vi "Circle dia adjust.vi"(8 "error in (no error)":errorcluster, 9 "Inspection \nmode?":bool, 10 "Cluster in":T1, 11 "Image in":T2) -> (0 "error out":errorcluster, 1 "Overlay Coordinates":cluster{"X":sgl, "Y":sgl}[](array[cluster]), 2 "Text origin":cluster{"X":sgl, "Y":sgl}, 3 "Image out":T2)   [LabVIEW 2019]
uses:
  <vilib>/vision/Image Controls.llb/IMAQ Image.ctl
  Controls/Circle dia data.ctl
  <vilib>/vision/NI_Vision_Development_Module.lvlib
panel:
  out "Angle":sgl
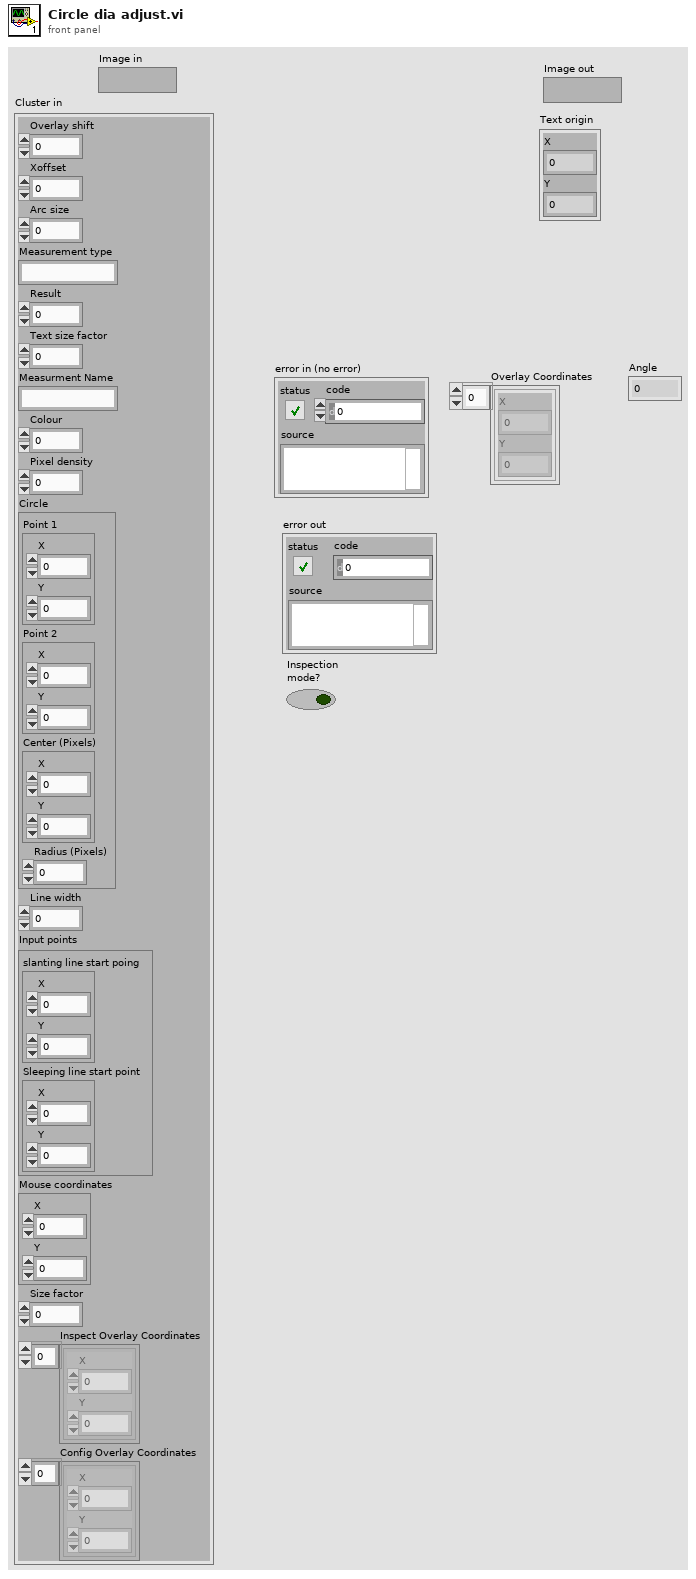
[diagram p1: front panel]
types:
  T1 = typedef "Circle dia data.ctl" = cluster{"Overlay shift":dbl, "Xoffset":i32, "Arc size":dbl, "Measurement type":string, "Result":sgl, "Text size factor":u32, "Measurment Name":string, "Colour":u32, "Pixel density":dbl, "Circle":cluster{"Point 1":cluster{"X":sgl, "Y":sgl}, "Point 2":cluster{"X":sgl, "Y":sgl}, "Center (Pixels)":cluster{"X":sgl, "Y":sgl}, "Radius (Pixels)":dbl}, "Line width":i32, "Input points":cluster{"slanting line start poing":cluster{"X":sgl, "Y":sgl}, "Sleeping line start point":cluster{"X":sgl, "Y":sgl}}, "Mouse coordinates":cluster{"X":sgl, "Y":sgl}, "Size factor":sgl, "Inspect Overlay Coordinates":cluster{"X":sgl, "Y":sgl}[], "Config Overlay Coordinates":cluster{"X":sgl, "Y":sgl}[]}
  T2 = typedef "IMAQ Image.ctl" = refnum<image>
  T3 = cluster{"Desired Font (Application)":enum16{"User-specified Font", "Application Font", "System Font", "Dialog Font"}, "[User-specified Font]":cluster{"Font Name":string, "Size":i16, "Strikeout?":bool, "Italic?":bool, "Underline?":bool, "Outline?":bool, "Shadow?":bool, "Bold?":bool, "Rotation Angle":dbl}, "Horizontal Alignment":i16, "Vertical Alignment":i16}
  T4 = cluster{"Left":i32, "Top":i32, "Right":i32, "Bottom":i32}
  T5 = cluster{"Point 1":cluster{"X":sgl, "Y":sgl}, "Point 2":cluster{"X":sgl, "Y":sgl}, "Center (Pixels)":cluster{"X":sgl, "Y":sgl}, "Radius (Pixels)":dbl}
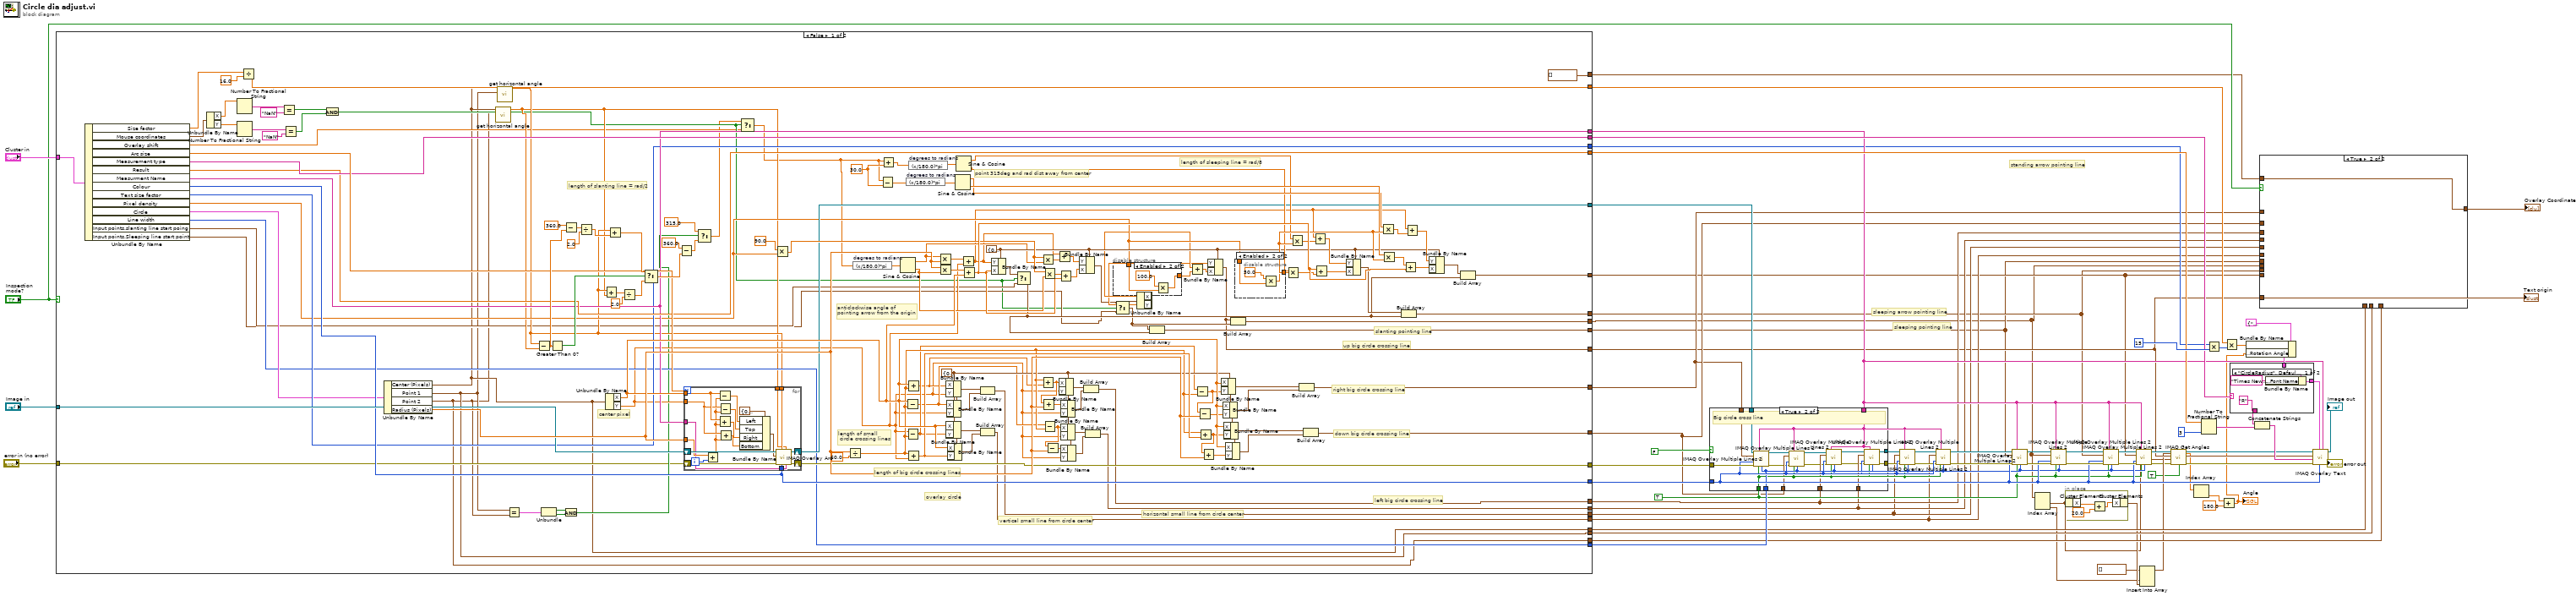
[diagram p0: block diagram]
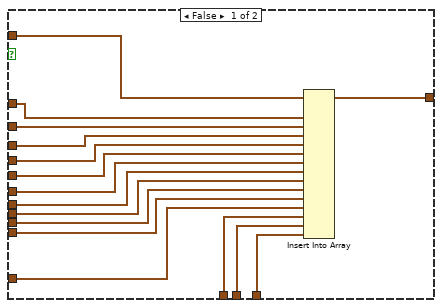
[diagram p2: hidden frame]
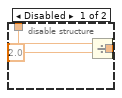
[diagram p3: hidden frame]
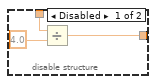
[diagram p4: hidden frame]
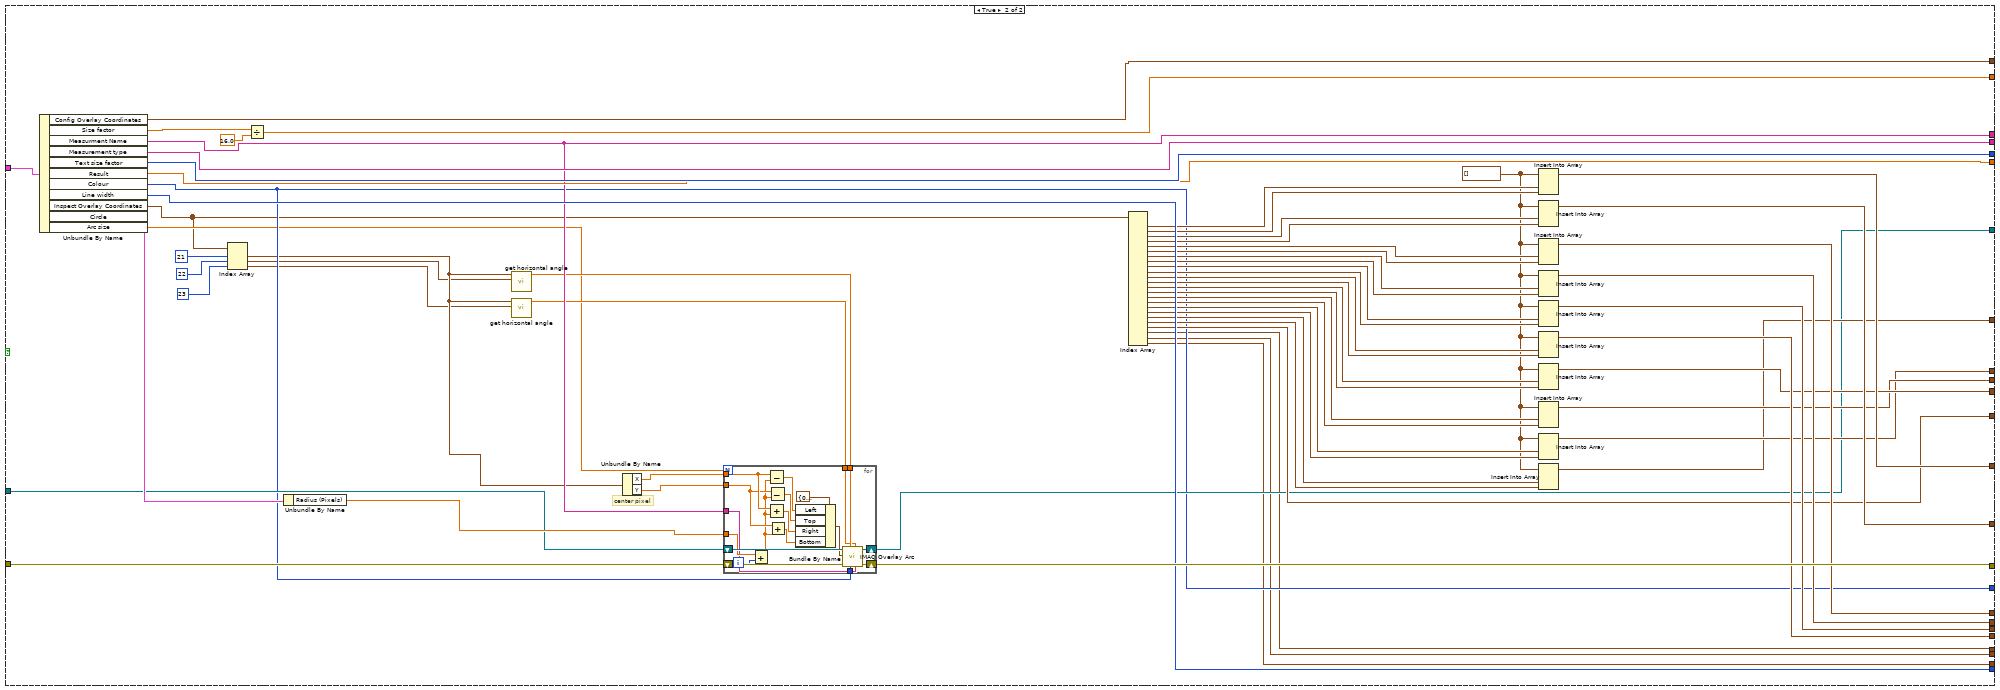
[diagram p5: hidden frame]
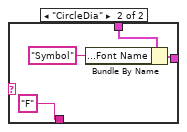
[diagram p7: hidden frame]
diagram:
  w38 = TRUE ("Maintain Width?")
  # "standing arrow pointing line"
  # "sleeping arrow pointing line"
  # "sleeping pointing line"
  n1 = case shown="False" "Inspection \nmode?" {
    tunnel: "error in (no error)" -> [w73 w298]
    tunnel: [w170 w298] -> w63
    tunnel: [w169 w252] -> w62
    tunnel: "Image in" -> [w168 w253]
    tunnel: "Cluster in" -> [w125 w301]
    tunnel: [w123 w296] -> w44
    tunnel: [w122 w293] -> w43
    tunnel: [w121 w256] -> w42
    tunnel: [w120 w251] -> w41
    tunnel: [w119 w295] -> w40
    tunnel: [w116 w294] -> w39
    tunnel: [w85 w297] -> w35
    tunnel: [w84 w269] -> w28
    tunnel: [w83 w268] -> w27
    tunnel: [w82 w267] -> w26
    tunnel: [w81 w266] -> w25
    tunnel: [w80 w270] -> w24
    tunnel: [w79 w271] -> w23
    tunnel: [w78 w263] -> w17
    tunnel: [w77 w264] -> w13
    tunnel: [w76 w265] -> w16
    tunnel: [w75 w261] -> w22
    tunnel: [w74 w262] -> w18
    tunnel: [w72 w249] -> w21
    tunnel: [w71 w248] -> w20
    tunnel: [w70 w247] -> w19
    tunnel: [cluster{"X":sgl, "Y":sgl}[] [] w239] -> w14
    frame False {
      w180 = 30.0 ("y")
      w164 = cluster{"X":sgl, "Y":sgl} {"X"=0.0, "Y"=0.0} ("Point 1")
      w146 = cluster{"X":sgl, "Y":sgl} {"X"=0.0, "Y"=0.0} ("Point 1")
      # "length of sleeping line = rad/8"
      # "point 315deg and rad dist away from center"
      # "length of slanting line = rad/2"
      # "length of small\n circle crossing lines"
      # "length of big circle crossing lines"
      # "anticlockwise angle of\npointing arrow from the origin"
      # "slanting pointing line"
      # "vertical small line from circle center"
      # "horizontal small line from circle center"
      # "left big circle crossing line"
      # "right big circle crossing line"
      # "down big circle crossing line"
      # "up big circle crossing line"
      # "center pixel"
      # "overlay circle"
      n2 = Unbundle By Name(w125) -> ("Size factor"=w87:sgl, "Mouse coordinates"=w97:cluster{"X":sgl, "Y":sgl}, "Overlay shift"=w99:dbl, "Arc size"=w124:dbl, "Measurement type"=w123:string, "Result"=w122:sgl, "Measurment Name"=w121:string, "Colour"=w120:u32, "Text size factor"=w119:u32, "Pixel density"=w118:dbl, "Circle"=w117:T5, "Line width"=w116:i32, "Input points.slanting line start poing"=w104:cluster{"X":sgl, "Y":sgl}, "Input points.Sleeping line start point"=w101:cluster{"X":sgl, "Y":sgl})
      n3 = Unbundle By Name(w97) -> ("X"=w96:sgl, "Y"=w95:sgl)
      n4 = Number To Fractional String(number=w96) -> (F-format string=w94:string)  [unwired: 3 in]
      n5 = Number To Fractional String(number=w95) -> (F-format string=w92:string)  [unwired: 3 in]
      n6 = Divide(x=w87, y=sgl 16.0) -> (x/y=w85:sgl)
      n7 = Equal?(x=w94, y="NaN") -> (x = y?=w90:bool)
      n8 = Equal?(x=w92, y="NaN") -> (x = y?=w89:bool)
      n9 = And(x=w90, y=w89) -> (x .and. y?=w100:bool)
      n10 = Unbundle By Name(w117) -> ("Center (Pixels)"=w72:cluster{"X":sgl, "Y":sgl}, "Point 1"=w71:cluster{"X":sgl, "Y":sgl}, "Point 2"=w70:cluster{"X":sgl, "Y":sgl}, "Radius (Pixels)"=w174:dbl)
      n11 = call "get horizontal angle.vi"("Point 2"=w70, "Point 1"=w72) -> ("Angle w.r.t horizontal\n(in degrees)"=w110:sgl)  [unwired: 9 in]
      n12 = call "get horizontal angle.vi"("Point 2"=w71, "Point 1"=w72) -> ("Angle w.r.t horizontal\n(in degrees)"=w111:sgl)  [unwired: 9 in]
      n13 = Equal?(x=w71, y=w70) -> (x = y?=w175:cluster{"X":bool, "Y":bool})
      n14 = Subtract(x=w111, y=w110) -> (x-y=w205:sgl)
      n15 = Unbundle(w175) -> ("X"=w176:bool, "Y"=w177:bool)
      n16 = Greater Than 0?(x=w205) -> (x > 0?=w202:bool)
      n17 = Subtract(x=sgl 360.0, y=w205) -> (x-y=w199:sgl)
      n18 = And(x=w176, y=w177) -> (x .and. y?=w106:bool)
      n19 = Divide(x=w199, y=sgl 2.0) -> (x/y=w201:sgl)
      n20 = Add(x=w111, y=w110) -> (x+y=w178:sgl)
      n21 = Unbundle By Name(w72) -> ("X"=w171:sgl, "Y"=w114:sgl)
      n22 = Add(x=w111, y=w201) -> (x+y=w204:sgl)
      n23 = Divide(x=w178, y=sgl 2.0) -> (x/y=w203:sgl)
      n24 = Select(t=w204, s=w202, f=w203) -> (s? t:f=w206:sgl)
      n25 = Subtract(x=sgl 360.0, y=w206) -> (x-y=w108:sgl)
      n26 = for {
        N: w124 -> [_]
        tunnel: w120 -> [w234]
        tunnel: w171 -> [w229]
        tunnel: w114 -> [w227]
        tunnel: w174 -> [w224]
        shift-right: [w237] -> w170
        shift-left: w73 -> [w238]
        shift-right: [w235] -> w169
        shift-left: w168 -> [w236]
        tunnel: w121 -> [w222]
        tunnel: w111 -> [w221]
        tunnel: w110 -> [w220]
        i -> [w225]
        n27 = Add(x=w224, y=w225) -> (x+y=w223:dbl)
        n28 = Subtract(x=w229, y=w223) -> (x-y=w231:dbl)
        n29 = Add(x=w229, y=w223) -> (x+y=w228:dbl)
        n30 = Subtract(x=w227, y=w223) -> (x-y=w230:dbl)
        n31 = Add(x=w227, y=w223) -> (x+y=w226:dbl)
        n32 = Bundle By Name(cluster=T4 {"Left"=0, "Top"=0, "Right"=0, "Bottom"=0} ("Bounding Rectangle"), "Left"=w231, "Top"=w230, "Right"=w228, "Bottom"=w226) -> (w232:T4)
        n33 = call "IMAQ Overlay Arc"("Group"=w222, "End Angle (degrees)"=w220, "Color"=w234, "Start Angle (degrees)"=w221, "error in (no error)"=w238, "Bounding Rectangle"=w232, "Image"=w236) -> ("error out"=w237:errorcluster, "Image Out"=w235:T2)  [unwired: 3 in]
      }
      n34 = Select(t=315.0, s=w106, f=w108) -> (s? t:f=w98:dbl)
      n35 = Select(t=w98, s=w100, f=w99) -> (s? t:f=w109:dbl)
      n36 = Multiply(x=sgl 90.0, y=w118) -> (x*y=w173:dbl)
      n37 = Divide(x=w174, y=sgl 60.0) -> (x/y=w151:dbl)
      n38 = expression code="(x/180.0)*pi" "degrees to radians"(w109) -> (w153:dbl)
      n39 = Subtract(x=w109, y=w180) -> (x-y=w182:dbl)
      n40 = Add(x=w109, y=w180) -> (x+y=w181:dbl)
      n41 = Sine & Cosine(0:w153) -> (1:w154:dbl, 2:w155:dbl)
      n42 = Subtract(x=w171, y=w151) -> (x-y=w138:dbl)
      n43 = Subtract(x=w114, y=w151) -> (x-y=w141:dbl)
      n44 = expression code="(x/180.0)*pi" "degrees to radians"(w182) -> (w184:dbl)
      n45 = Add(x=w171, y=w151) -> (x+y=w131:dbl)
      n46 = Add(x=w151, y=w114) -> (x+y=w152:dbl)
      n47 = expression code="(x/180.0)*pi" "degrees to radians"(w181) -> (w183:dbl)
      n48 = Multiply(x=w154, y=w174) -> (x*y=w166:dbl)
      n49 = Multiply(x=w174, y=w155) -> (x*y=w167:dbl)
      n50 = Bundle By Name(cluster=w146, "X"=w131, "Y"=w114) -> (w126:cluster{"X":sgl, "Y":sgl})
      n51 = Bundle By Name(cluster=w146, "X"=w171, "Y"=w141) -> (w128:cluster{"X":sgl, "Y":sgl})
      n52 = Bundle By Name(cluster=w146, "X"=w138, "Y"=w114) -> (w127:cluster{"X":sgl, "Y":sgl})
      n53 = Bundle By Name(cluster=w146, "X"=w171, "Y"=w152) -> (w129:cluster{"X":sgl, "Y":sgl})
      n54 = Sine & Cosine(0:w184) -> (1:w190:dbl, 2:w191:dbl)
      n55 = Sine & Cosine(0:w183) -> (1:w187:dbl, 2:w185:dbl)
      n56 = Add(x=w166, y=w114) -> (x+y=w115:dbl)
      n57 = Add(x=w167, y=w171) -> (x+y=w196:dbl)
      n58 = Build Array(w126, w127) -> (w82:cluster{"X":sgl, "Y":sgl}[])
      n59 = Build Array(w128, w129) -> (w81:cluster{"X":sgl, "Y":sgl}[])
      n60 = Bundle By Name(cluster=w164, "Y"=w115, "X"=w196) -> (w105:cluster{"X":sgl, "Y":sgl})
      n61 = Select(t=w105, s=w100, f=w104) -> (s? t:f=w103:cluster{"X":sgl, "Y":sgl})
      n62 = Multiply(x=w173, y=w154) -> (x*y=w156:dbl)
      n63 = Add(x=w151, y=w131) -> (x+y=w133:dbl)
      n64 = Add(x=w133, y=w174) -> (x+y=w132:dbl)
      n65 = Multiply(x=w173, y=w155) -> (x*y=w157:dbl)
      n66 = Subtract(x=w138, y=w151) -> (x-y=w137:dbl)
      n67 = Subtract(x=w137, y=w174) -> (x-y=w136:dbl)
      n68 = Add(x=w115, y=w156) -> (x+y=w161:dbl)
      n69 = Add(x=w157, y=w196) -> (x+y=w162:dbl)
      n70 = Bundle By Name(cluster=w146, "X"=w133, "Y"=w114) -> (w134:cluster{"X":sgl, "Y":sgl})
      n71 = Bundle By Name(cluster=w146, "X"=w132, "Y"=w114) -> (w135:cluster{"X":sgl, "Y":sgl})
      n72 = Bundle By Name(cluster=w146, "X"=w137, "Y"=w114) -> (w139:cluster{"X":sgl, "Y":sgl})
      n73 = Bundle By Name(cluster=w146, "X"=w136, "Y"=w114) -> (w140:cluster{"X":sgl, "Y":sgl})
      n74 = Bundle By Name(cluster=w164, "Y"=w161, "X"=w162) -> (w102:cluster{"X":sgl, "Y":sgl})
      n75 = Build Array(w134, w135) -> (w84:cluster{"X":sgl, "Y":sgl}[])
      n76 = Build Array(w139, w140) -> (w83:cluster{"X":sgl, "Y":sgl}[])
      n77 = disable-structure shown="Enabled" {
        disable-tunnel: [w215 w217] -> w158
        disable-tunnel: w118 -> [w214 w219]
        frame Disabled {
          n78 = Divide(x=w214, y=4.0) -> (x/y=w215:dbl)
        }
        frame Enabled {
          n79 = Multiply(x=100.0, y=w219) -> (x*y=w217:dbl)
        }
      }
      n80 = Select(t=w102, s=w100, f=w101) -> (s? t:f=w88:cluster{"X":sgl, "Y":sgl})
      n81 = Unbundle By Name(w88) -> ("X"=w113:sgl, "Y"=w112:sgl)
      n82 = Build Array(w88, w103) -> (w76:cluster{"X":sgl, "Y":sgl}[])
      n83 = Add(x=w113, y=w158) -> (x+y=w159:dbl)
      n84 = Subtract(x=w141, y=w151) -> (x-y=w143:dbl)
      n85 = Subtract(x=w143, y=w174) -> (x-y=w142:dbl)
      n86 = Add(x=w151, y=w152) -> (x+y=w148:dbl)
      n87 = Add(x=w148, y=w174) -> (x+y=w147:dbl)
      n88 = Bundle By Name(cluster=w164, "Y"=w112, "X"=w159) -> (w75:cluster{"X":sgl, "Y":sgl})
      n89 = Bundle By Name(cluster=w146, "X"=w171, "Y"=w143) -> (w144:cluster{"X":sgl, "Y":sgl})
      n90 = Bundle By Name(cluster=w146, "X"=w171, "Y"=w142) -> (w145:cluster{"X":sgl, "Y":sgl})
      n91 = Bundle By Name(cluster=w146, "X"=w171, "Y"=w148) -> (w149:cluster{"X":sgl, "Y":sgl})
      n92 = Bundle By Name(cluster=w146, "X"=w171, "Y"=w147) -> (w150:cluster{"X":sgl, "Y":sgl})
      n93 = Build Array(w75, w88) -> (w77:cluster{"X":sgl, "Y":sgl}[])
      n94 = disable-structure shown="Enabled" {
        disable-tunnel: w118 -> [w210 w212]
        disable-tunnel: [w208 w211] -> w192
        frame Disabled {
          n95 = Divide(x=w210, y=sgl 2.0) -> (x/y=w208:dbl)
        }
        frame Enabled {
          n96 = Multiply(x=sgl 50.0, y=w212) -> (x*y=w211:dbl)
        }
      }
      n97 = Multiply(x=w185, y=w192) -> (x*y=w186:dbl)
      n98 = Multiply(x=w187, y=w192) -> (x*y=w188:dbl)
      n99 = Build Array(w144, w145) -> (w79:cluster{"X":sgl, "Y":sgl}[])
      n100 = Build Array(w149, w150) -> (w80:cluster{"X":sgl, "Y":sgl}[])
      n101 = Add(x=w115, y=w188) -> (x+y=w189:dbl)
      n102 = Add(x=w196, y=w186) -> (x+y=w160:dbl)
      n103 = Bundle By Name(cluster=w164, "Y"=w189, "X"=w160) -> (w163:cluster{"X":sgl, "Y":sgl})
      n104 = Multiply(x=w190, y=w192) -> (x*y=w193:dbl)
      n105 = Multiply(x=w191, y=w192) -> (x*y=w195:dbl)
      n106 = Build Array(w163, w103) -> (w78:cluster{"X":sgl, "Y":sgl}[])
      n107 = Add(x=w195, y=w196) -> (x+y=w197:dbl)
      n108 = Add(x=w115, y=w193) -> (x+y=w194:dbl)
      n109 = Bundle By Name(cluster=w164, "Y"=w194, "X"=w197) -> (w165:cluster{"X":sgl, "Y":sgl})
      n110 = Build Array(w165, w103) -> (w74:cluster{"X":sgl, "Y":sgl}[])
    }
    frame True {
      w272 = cluster{"X":sgl, "Y":sgl}[] [] ("array")
      # "center pixel"
      n111 = Unbundle By Name(w301) -> ("Config Overlay Coordinates"=w239:cluster{"X":sgl, "Y":sgl}[], "Size factor"=w299:sgl, "Measurment Name"=w256:string, "Measurement type"=w296:string, "Text size factor"=w295:u32, "Result"=w293:sgl, "Colour"=w251:u32, "Line width"=w294:i32, "Inspect Overlay Coordinates"=w240:cluster{"X":sgl, "Y":sgl}[], "Circle"=w257:T5, "Arc size"=w250:dbl)
      n112 = Index Array(array=w240, index #1=21 ("index"), index #2=22 ("index"), index #3=23 ("index")) -> (element #1=w243:cluster{"X":sgl, "Y":sgl}, element #2=w242:cluster{"X":sgl, "Y":sgl}, element #3=w241:cluster{"X":sgl, "Y":sgl})
      n113 = Divide(x=w299, y=sgl 16.0) -> (x/y=w297:sgl)
      n114 = Unbundle By Name(w257) -> ("Radius (Pixels)"=w260:dbl)
      n115 = call "get horizontal angle.vi"("Point 2"=w242, "Point 1"=w243) -> ("Angle w.r.t horizontal\n(in degrees)"=w254:sgl)  [unwired: 9 in]
      n116 = call "get horizontal angle.vi"("Point 2"=w241, "Point 1"=w243) -> ("Angle w.r.t horizontal\n(in degrees)"=w255:sgl)  [unwired: 9 in]
      n117 = Unbundle By Name(w243) -> ("X"=w259:sgl, "Y"=w258:sgl)
      n118 = for {
        N: w250 -> [_]
        tunnel: w251 -> [w316]
        tunnel: w259 -> [w311]
        tunnel: w258 -> [w309]
        tunnel: w260 -> [w306]
        shift-right: [w319] -> _
        shift-left: _ -> [w320]
        shift-right: [w317] -> w252
        shift-left: w253 -> [w318]
        tunnel: w256 -> [w304]
        tunnel: w254 -> [w303]
        tunnel: w255 -> [w302]
        i -> [w307]
        n119 = Add(x=w306, y=w307) -> (x+y=w305:dbl)
        n120 = Subtract(x=w311, y=w305) -> (x-y=w313:dbl)
        n121 = Add(x=w311, y=w305) -> (x+y=w310:dbl)
        n122 = Subtract(x=w309, y=w305) -> (x-y=w312:dbl)
        n123 = Add(x=w309, y=w305) -> (x+y=w308:dbl)
        n124 = Bundle By Name(cluster=T4 {"Left"=0, "Top"=0, "Right"=0, "Bottom"=0} ("Bounding Rectangle"), "Left"=w313, "Top"=w312, "Right"=w310, "Bottom"=w308) -> (w314:T4)
        n125 = call "IMAQ Overlay Arc"("Group"=w304, "End Angle (degrees)"=w302, "Color"=w316, "Start Angle (degrees)"=w303, "error in (no error)"=w320, "Bounding Rectangle"=w314, "Image"=w318) -> ("error out"=w319:errorcluster, "Image Out"=w317:T2)  [unwired: 3 in]
      }
      n126 = Index Array(array=w240) -> (element #1=w292:cluster{"X":sgl, "Y":sgl}, element #2=w291:cluster{"X":sgl, "Y":sgl}, element #3=w290:cluster{"X":sgl, "Y":sgl}, element #4=w289:cluster{"X":sgl, "Y":sgl}, element #5=w288:cluster{"X":sgl, "Y":sgl}, element #6=w287:cluster{"X":sgl, "Y":sgl}, element #7=w286:cluster{"X":sgl, "Y":sgl}, element #8=w285:cluster{"X":sgl, "Y":sgl}, element #9=w284:cluster{"X":sgl, "Y":sgl}, element #10=w283:cluster{"X":sgl, "Y":sgl}, element #11=w282:cluster{"X":sgl, "Y":sgl}, element #12=w281:cluster{"X":sgl, "Y":sgl}, element #13=w280:cluster{"X":sgl, "Y":sgl}, element #14=w279:cluster{"X":sgl, "Y":sgl}, element #15=w278:cluster{"X":sgl, "Y":sgl}, element #16=w277:cluster{"X":sgl, "Y":sgl}, element #17=w276:cluster{"X":sgl, "Y":sgl}, element #18=w275:cluster{"X":sgl, "Y":sgl}, element #19=w274:cluster{"X":sgl, "Y":sgl}, element #20=w273:cluster{"X":sgl, "Y":sgl}, element #21=w261:cluster{"X":sgl, "Y":sgl}, element #22=w249:cluster{"X":sgl, "Y":sgl}, element #23=w248:cluster{"X":sgl, "Y":sgl}, element #24=w247:cluster{"X":sgl, "Y":sgl})  [unwired: 24 in]
      n127 = Insert Into Array(array=w272, new element #1=w292, new element #2=w291) -> (w271:cluster{"X":sgl, "Y":sgl}[])  [unwired: 1 in]
      n128 = Insert Into Array(array=w272, new element #1=w290, new element #2=w289) -> (w270:cluster{"X":sgl, "Y":sgl}[])  [unwired: 1 in]
      n129 = Insert Into Array(array=w272, new element #1=w288, new element #2=w287) -> (w269:cluster{"X":sgl, "Y":sgl}[])  [unwired: 1 in]
      n130 = Insert Into Array(array=w272, new element #1=w286, new element #2=w285) -> (w268:cluster{"X":sgl, "Y":sgl}[])  [unwired: 1 in]
      n131 = Insert Into Array(array=w272, new element #1=w284, new element #2=w283) -> (w267:cluster{"X":sgl, "Y":sgl}[])  [unwired: 1 in]
      n132 = Insert Into Array(array=w272, new element #1=w282, new element #2=w281) -> (w266:cluster{"X":sgl, "Y":sgl}[])  [unwired: 1 in]
      n133 = Insert Into Array(array=w272, new element #1=w280, new element #2=w279) -> (w265:cluster{"X":sgl, "Y":sgl}[])  [unwired: 1 in]
      n134 = Insert Into Array(array=w272, new element #1=w278, new element #2=w277) -> (w264:cluster{"X":sgl, "Y":sgl}[])  [unwired: 1 in]
      n135 = Insert Into Array(array=w272, new element #1=w276, new element #2=w275) -> (w263:cluster{"X":sgl, "Y":sgl}[])  [unwired: 1 in]
      n136 = Insert Into Array(array=w272, new element #1=w274, new element #2=w273) -> (w262:cluster{"X":sgl, "Y":sgl}[])  [unwired: 1 in]
    }
  }
  "Text origin" <- w22
  n137 = case shown="True" FALSE {
    tunnel: w63 -> [w321 w340]
    tunnel: w62 -> [w322 w339]
    tunnel: w23 -> [_ w338]
    tunnel: w24 -> [_ w337]
    tunnel: w28 -> [_ w336]
    tunnel: w27 -> [_ w335]
    tunnel: w42 -> [_ w334]
    tunnel: w41 -> [_ w333]
    tunnel: w39 -> [_ w332]
    tunnel: w38 -> [_ w331]
    tunnel: [w321 w326] -> w34
    tunnel: [w322 w323] -> w32
    frame False {
    }
    frame True {
      # "Big circle cross line"
      n138 = call "IMAQ Overlay Multiple Lines 2"("Image"=w339, "Group"=w334, "Line End Points"=w338, "Color"=w333, "error in (no error)"=w340, "Maintain Width?"=w331, "Width"=w332) -> ("Image Out"=w330:T2, "error out"=w329:errorcluster)  [unwired: 7 in]
      n139 = call "IMAQ Overlay Multiple Lines 2"("Image"=w330, "Group"=w334, "Line End Points"=w337, "Color"=w333, "error in (no error)"=w329, "Maintain Width?"=w331, "Width"=w332) -> ("Image Out"=w325:T2, "error out"=w328:errorcluster)  [unwired: 7 in]
      n140 = call "IMAQ Overlay Multiple Lines 2"("Image"=w325, "Group"=w334, "Line End Points"=w336, "Color"=w333, "error in (no error)"=w328, "Maintain Width?"=w331, "Width"=w332) -> ("Image Out"=w324:T2, "error out"=w327:errorcluster)  [unwired: 7 in]
      n141 = call "IMAQ Overlay Multiple Lines 2"("Image"=w324, "Group"=w334, "Line End Points"=w335, "Color"=w333, "error in (no error)"=w327, "Maintain Width?"=w331, "Width"=w332) -> ("Image Out"=w323:T2, "error out"=w326:errorcluster)  [unwired: 7 in]
    }
  }
  n142 = call "IMAQ Overlay Multiple Lines 2"("Image"=w32, "Group"=w42, "Line End Points"=w26, "Color"=w41, "error in (no error)"=w34, "Maintain Width?"=w38, "Width"=w39) -> ("Image Out"=w31:T2, "error out"=w33:errorcluster)  [unwired: 7 in]
  n143 = call "IMAQ Overlay Multiple Lines 2"("Image"=w31, "Group"=w42, "Line End Points"=w25, "Color"=w41, "error in (no error)"=w33, "Maintain Width?"=w38, "Width"=w39) -> ("Image Out"=w49:T2, "error out"=w46:errorcluster)  [unwired: 7 in]
  n144 = call "IMAQ Overlay Multiple Lines 2"("Image"=w49, "Group"=w42, "Line End Points"=w16, "Color"=w41, "error in (no error)"=w46, "Maintain Width?"=w38, "Width"=w39) -> ("Image Out"=w48:T2, "error out"=w47:errorcluster)  [unwired: 7 in]
  n145 = Index Array(array=w13) -> (element #1=w5:cluster{"X":sgl, "Y":sgl}, element #2=w4:cluster{"X":sgl, "Y":sgl})  [unwired: 2 in]
  n146 = call "IMAQ Overlay Multiple Lines 2"("Image"=w48, "Group"=w42, "Line End Points"=w13, "Color"=w41, "error in (no error)"=w47, "Maintain Width?"=w38, "Width"=w39) -> ("Image Out"=w51:T2, "error out"=w50:errorcluster)  [unwired: 7 in]
  n147 = in-place {
    n148 = in-place-cluster #1(w5) -> ("X"=w343:sgl)
    n149 = Add(x=w343, y=sgl 20.0) -> (x+y=w342:sgl)
    n150 = in-place-cluster #1("X"=w342) -> (w12:cluster{"X":sgl, "Y":sgl})
  }
  n151 = call "IMAQ Overlay Multiple Lines 2"("Image"=w51, "Group"=w42, "Line End Points"=w17, "Color"=w41, "error in (no error)"=w50, "Maintain Width?"=w38, "Width"=w39) -> ("Image Out"=w52:T2, "error out"=w53:errorcluster)  [unwired: 7 in]
  n152 = call "IMAQ Overlay Multiple Lines 2"("Image"=w52, "Group"=w42, "Line End Points"=w18, "Color"=w41, "error in (no error)"=w53, "Maintain Width?"=w38, "Width"=w39) -> ("Image Out"=w55:T2, "error out"=w9:errorcluster)  [unwired: 7 in]
  n153 = Insert Into Array(array=cluster{"X":sgl, "Y":sgl}[] [], new element #1=w4, new element #2=w12) -> (w11:cluster{"X":sgl, "Y":sgl}[])  [unwired: 1 in]
  n154 = call "IMAQ Get Angles"("error in (no error)"=w9, "Vertex"=w5, "Points"=w11, "Use Vertex (No)"=TRUE) -> ("error out"=w8:errorcluster, "Angles (deg)"=w7:sgl[])  [unwired: 1 in, 1 out]
  n155 = Index Array(array=w7) -> (element=w3:sgl)  [unwired: 1 in]
  n156 = Number To Fractional String(number=w43, precision (6)=i16 3) -> (F-format string=w60:string)  [unwired: 2 in]
  n157 = Multiply(x=w40, y=15) -> (x*y=w36:u32)
  n158 = Add(x=w3, y=sgl 180.0) -> (x+y=w1:sgl)
  "Angle" <- w1
  n159 = Multiply(x=w35, y=w36) -> (x*y=w37:sgl)
  n160 = Bundle By Name(cluster=T3 {"Desired Font (Application)"=enum."User-specified Font", "[User-specified Font]"={"Font Name"="Symbol", "Size"=130, "Strikeout?"=FALSE, "Italic?"=FALSE, "Underline?"=FALSE, "Outline?"=FALSE, "Shadow?"=FALSE, "Bold?"=TRUE, "Rotation Angle"=0.0}, "Horizontal Alignment"=0, "Vertical Alignment"=2} ("Font, Size & Style"), "[User-specified Font].Size"=w37, "[User-specified Font].Rotation Angle"=w1) -> (w67:T3)
  n161 = case shown="\"CircleRadius\", Default" w44 {
    tunnel: ["R" "F" ("string")] -> w59
    tunnel: w67 -> [w346 w350]
    tunnel: [w345 w349] -> w68
    frame "CircleRadius", Default {
      n162 = Bundle By Name(cluster=w346, "[User-specified Font].Font Name"="Times New Roman") -> (w345:T3)
    }
    frame "CircleDia" {
      n163 = Bundle By Name(cluster=w350, "[User-specified Font].Font Name"="Symbol") -> (w349:T3)
    }
  }
  n164 = Concatenate Strings(w59, w60) -> (w58:string)
  n165 = case shown="True" "Inspection \nmode?" {
    tunnel: [w367 w368] -> w29
    tunnel: w28 -> [w366 _]
    tunnel: w27 -> [w365 _]
    tunnel: w26 -> [w364 _]
    tunnel: w25 -> [w363 _]
    tunnel: w24 -> [w362 _]
    tunnel: w23 -> [w361 _]
    tunnel: w22 -> [w360 _]
    tunnel: w21 -> [w359 _]
    tunnel: w20 -> [w358 _]
    tunnel: w19 -> [w357 _]
    tunnel: w18 -> [w356 _]
    tunnel: w17 -> [w355 _]
    tunnel: w16 -> [w354 _]
    tunnel: w13 -> [w353 _]
    tunnel: w14 -> [w352 w368]
    frame False {
      n166 = Insert Into Array(array=w352, new element #1=w361, new element #2=w362, new element #3=w366, new element #4=w365, new element #5=w364, new element #6=w363, new element #7=w354, new element #8=w353, new element #9=w355, new element #10=w356, new element #11=w360, new element #12=w359, new element #13=w358, new element #14=w357) -> (w367:cluster{"X":sgl, "Y":sgl}[])  [unwired: 1 in]
    }
    frame True {
    }
  }
  "Overlay Coordinates" <- w29
  n167 = call "IMAQ Overlay Text"("Group"=w42, "Text Color (black)"=w41, "Font, Size & Style"=w68, "error in (no error)"=w8, "String"=w58, "Origin"=w22, "Image"=w55) -> ("error out"=→"error out":errorcluster, "Image Out"=→"Image out":T2)  [unwired: 3 in]
